vi "to string.vi"(8 "error in":errorcluster, 11 "configuration in":refnum<class "PL_Target Configuration.lvclass">) -> (0 "error out":errorcluster, 1 "data":string, 2 "version":string, 3 "configuration out":refnum<class "PL_Target Configuration.lvclass">)   [LabVIEW 2013, in "PL_Target Configuration.lvclass"]
doc: "Provides an interface for saving a module configuration to a file or other serialized data source. It is recommended that all children of this class store data in two sets--data required for its own initialization, and any data required for parent initialization--and that each implementation uses the <b>Call Parent Method</b> primitive to serialize parent information."
uses:
  PL_Target Configuration.lvclass
  <vilib>/NI/Tag Bus Module Framework/root configuration/TBM configuration.lvclass
  PL_Target Configuration.lvclass/PL_Target Configuration.ctl
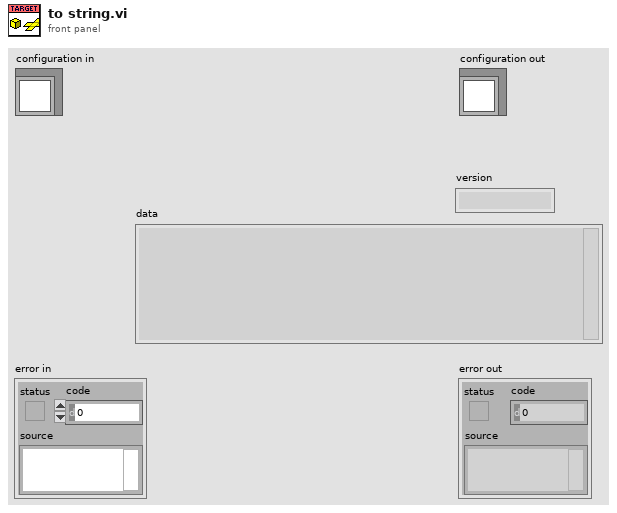
[diagram p1: front panel]
types:
  T1 = typedef "TBM configuration.lvclass/Target Types.ctl" = enum16{"Windows", "Mac", "Linux", "Linux RT ARM", "VxWorks", "Pharlap", "Other", "Linux RT x64"}
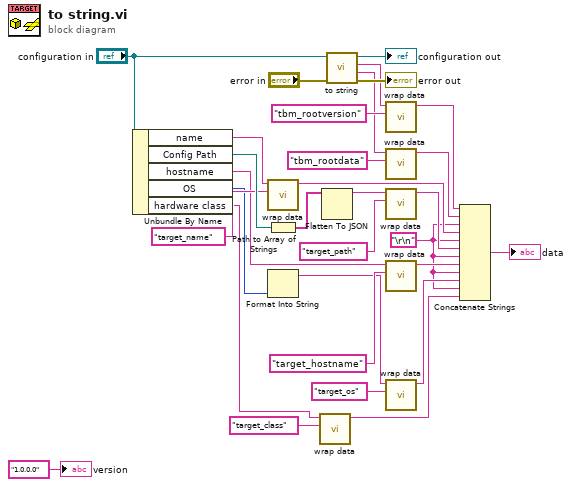
[diagram p0: block diagram]
diagram:
  w1 = "\r\n"
  n1 = Unbundle By Name("configuration in") -> ("name"=w22:string, "Config Path"=w21:path, "hostname"=w11:string, "OS"=w7:T1, "hardware class"=w6:string)
  n2 = call <vilib>:"wrap data.vi"("identifier"="target_name" ("additional identifier"), "data to wrap"=w22) -> ("wrapped data"=w16:string)  [unwired: 9 in]
  n3 = Path to Array of Strings(0:w21) -> (2:w20:string[])  [unwired: 1 out]
  n4 = Format Into String(w7) -> (resulting string=w4:string)  [unwired: 3 in, 1 out]
  n5 = call <vilib>:"wrap data.vi"("identifier"="target_class" ("additional identifier"), "data to wrap"=w6) -> ("wrapped data"=w3:string)  [unwired: 9 in]
  n6 = Flatten To JSON(anything=w20) -> (JSON string=w19:string)  [unwired: 2 in, 1 out]
  n7 = call-parent "to string.vi"("error in"="error in", "configuration in"="configuration in") -> ("error out"=→"error out":errorcluster, "data"=w24:string, "version"=w25:string, "configuration out"=→"configuration out":refnum<class "PL_Target Configuration.lvclass">)  [unwired: 6 in]
  n8 = call <vilib>:"wrap data.vi"("identifier"="tbm_rootversion" ("additional identifier"), "data to wrap"=w25) -> ("wrapped data"=w18:string)  [unwired: 9 in]
  n9 = call <vilib>:"wrap data.vi"("identifier"="tbm_rootdata" ("additional identifier"), "data to wrap"=w24) -> ("wrapped data"=w17:string)  [unwired: 9 in]
  n10 = call <vilib>:"wrap data.vi"("identifier"="target_path" ("additional identifier"), "data to wrap"=w19) -> ("wrapped data"=w15:string)  [unwired: 9 in]
  n11 = call <vilib>:"wrap data.vi"("identifier"="target_hostname" ("additional identifier"), "data to wrap"=w11) -> ("wrapped data"=w9:string)  [unwired: 9 in]
  n12 = call <vilib>:"wrap data.vi"("identifier"="target_os" ("additional identifier"), "data to wrap"=w4) -> ("wrapped data"=w2:string)  [unwired: 9 in]
  n13 = Concatenate Strings(w18, w17, w1, w16, w1, w15, w1, w9, w1, w2, w1, w3) -> (→"data":string)
  "version" <- "1.0.0.0" ("version")
